vi "Meas Result Get Readings.vi"(5 "table ref":refnum<vi>, 8 "error in (no error)":errorcluster, 9 "ring spot":refnum<vi>, 10 "ring phase":refnum<vi>, 11 "result":T3) -> (0 "error out":errorcluster, 1 "sweep spot index":u16, 2 "phase index":u16, 3 "readings":T1, 4 "quantities":T2)   [LabVIEW 2020]
doc: "Gets readings for selected sweep spot."
uses:
  Meas Results.ctl
  bridge/Bridge Frequency Readings Data.ctl
  drivers/TWM client/Meas Proc QWTB Spectrum Data.ctl
  drivers/TWM client/TWM Phase Info.ctl
  Meas Quantity Names.ctl
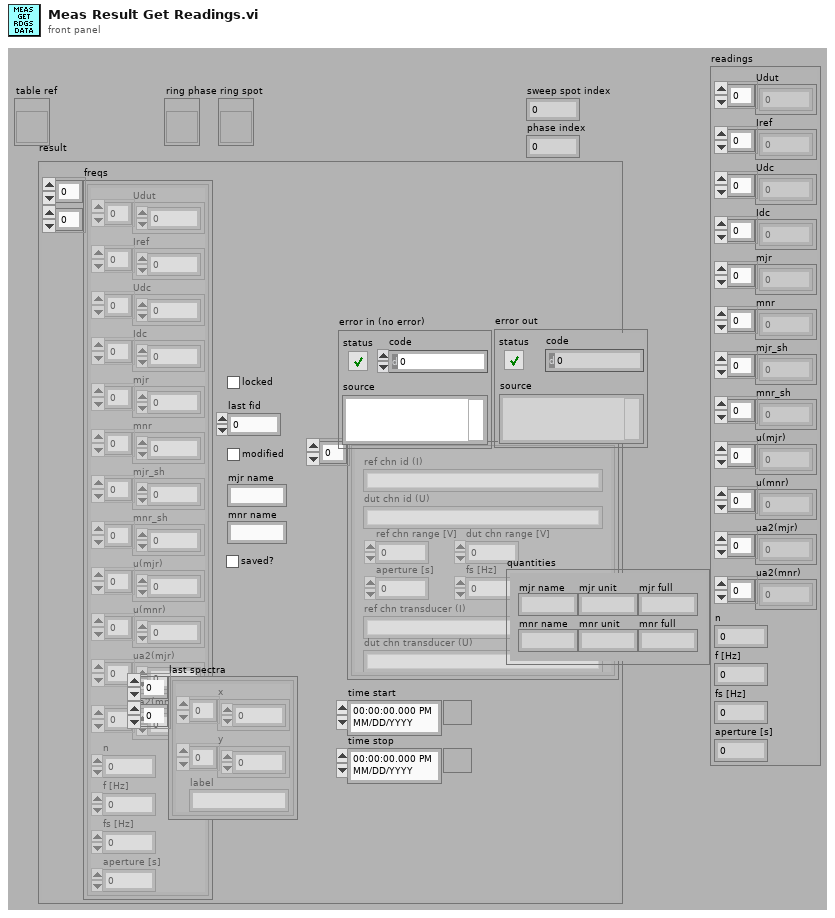
[diagram p1: front panel]
types:
  T1 = typedef "Bridge Frequency Readings Data.ctl" = cluster{"Udut":dbl[], "Iref":dbl[], "Udc":dbl[], "Idc":dbl[], "mjr":dbl[], "mnr":dbl[], "mjr_sh":dbl[], "mnr_sh":dbl[], "u(mjr)":dbl[], "u(mnr)":dbl[], "ua2(mjr)":dbl[], "ua2(mnr)":dbl[], "n":i32, "f [Hz]":dbl, "fs [Hz]":dbl, "aperture [s]":dbl}
  T2 = typedef "Meas Quantity Names.ctl" = cluster{"mjr name":string, "mnr name":string, "mjr unit":string, "mnr unit":string, "mjr full":string, "mnr full":string}
  T3 = typedef "Meas Results.ctl" = cluster{"freqs":T1[][], "locked":bool, "last fid":i32, "modified":bool, "mjr name":string, "mnr name":string, "last spectra":T4[][], "saved?":bool, "TWM phase":T5[], "time start":timestamp, "time stop":timestamp}
  T4 = typedef "Meas Proc QWTB Spectrum Data.ctl" = cluster{"x":sgl[], "y":sgl[], "label":string}
  T5 = typedef "TWM Phase Info.ctl" = cluster{"ref chn id (I)":string, "dut chn id (U)":string, "ref chn range [V]":dbl, "dut chn range [V]":dbl, "aperture [s]":dbl, "fs [Hz]":dbl, "ref chn transducer (I)":string, "dut chn transducer (U)":string}
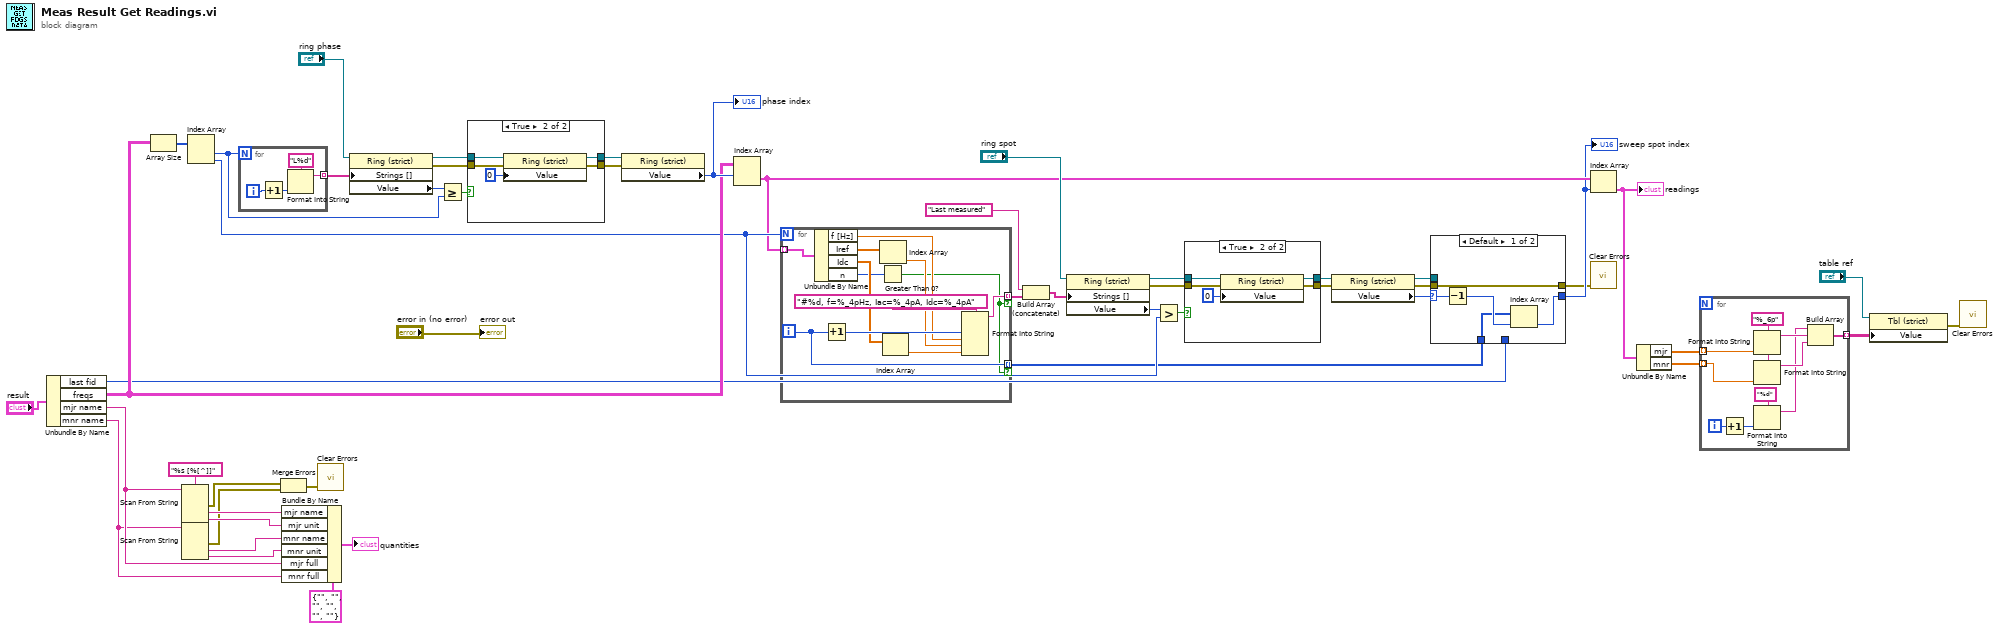
[diagram p0: block diagram]
diagram:
  w47 = "%s [%[^]]" ("format string")
  n1 = Unbundle By Name("result") -> ("last fid"=w3:i32, "freqs"=w27:T1[][], "mjr name"=w44:string, "mnr name"=w43:string)
  n2 = Array Size(array=w27) -> (size(s)=w38:i32[])
  n3 = Scan From String(format string=w47, input string=w44) -> (error out=w40:errorcluster, output 1=w49:string, output 2=w48:string)  [unwired: 4 in, 2 out]
  n4 = Scan From String(format string=w47, input string=w43) -> (error out=w41:errorcluster, output 1=w46:string, output 2=w45:string)  [unwired: 4 in, 2 out]
  n5 = Index Array(array=w38) -> (element #1=w34:i32, element #2=w24:i32)  [unwired: 2 in]
  n6 = for {
    N: w34 -> [_]
    tunnel: [w52] -> w36 mode=indexing
    i -> [w53]
    n7 = Increment(x=w53) -> (x+1=w54:i32)
    n8 = Format Into String(format string="L%d", w54) -> (resulting string=w52:string)  [unwired: 2 in, 1 out]
  }
  n9 = Merge Errors(w40, w41) -> (w39:errorcluster)
  n10 = Bundle By Name(cluster=T2 {"mjr name"="", "mnr name"="", "mjr unit"="", "mnr unit"="", "mjr full"="", "mnr full"=""} ("quantities"), "mjr name"=w49, "mjr unit"=w48, "mnr name"=w46, "mnr unit"=w45, "mjr full"=w44, "mnr full"=w43) -> (→"quantities":T2)
  n11 = call <vilib>:"Clear Errors.vi"("error in (no error)"=w39) -> ()  [unwired: 5 in, 2 out]
  n12 = property class="Ring (strict)"(reference="ring phase", "Strings []"=w36) -> (reference out=w32:refnum<vi>, error out=w30:errorcluster, "Value"=w35:u16)  [unwired: 1 in]
  n13 = Greater Or Equal?(x=w35, y=w34) -> (x >= y?=w33:bool)
  n14 = case shown="True" w33 {
    tunnel: w32 -> [w57 w62]
    tunnel: [w57 w60] -> w31
    tunnel: [w56 w58] -> w29
    tunnel: w30 -> [w56 w59]
    frame False {
    }
    frame True {
      n15 = property class="Ring (strict)"(reference=w62, error in=w59, "Value"=u16 0) -> (reference out=w60:refnum<vi>, error out=w58:errorcluster)
    }
  }
  n16 = property class="Ring (strict)"(reference=w31, error in=w29) -> ("Value"=w28:u16)  [unwired: 2 out]
  "phase index" <- w28
  n17 = Index Array(array=w27, index (row)=w28) -> (element=w16:T1[])  [unwired: 1 in]
  n18 = for {
    N: w24 -> [_]
    tunnel: [w72] -> w8 mode=indexing if=w63
    tunnel: w16 -> [w71] mode=indexing
    tunnel: [w64] -> w1 mode=indexing if=w63
    i -> [w64]
    n19 = Unbundle By Name(w71) -> ("f [Hz]"=w70:dbl, "Iref"=w69:dbl[], "Idc"=w67:dbl[], "n"=w65:i32)
    n20 = Increment(x=w64) -> (x+1=w73:i32)
    n21 = Index Array(array=w69) -> (element=w68:dbl)  [unwired: 1 in]
    n22 = Greater Than 0?(x=w65) -> (x > 0?=w63:bool)
    n23 = Index Array(array=w67) -> (element=w66:dbl)  [unwired: 1 in]
    n24 = Format Into String(format string="#%d, f=%_4pHz, Iac=%_4pA, Idc=%_4pA", w73, w70, w68, w66) -> (resulting string=w72:string)  [unwired: 2 in, 1 out]
  }
  n25 = Build Array (concatenate)("Last measured", w8) -> (w7:string[])
  n26 = property class="Ring (strict)"(reference="ring spot", "Strings []"=w7) -> (reference out=w22:refnum<vi>, error out=w23:errorcluster, "Value"=w25:u16)  [unwired: 1 in]
  n27 = Greater?(x=w25, y=w24) -> (0:w21:bool)
  n28 = case shown="True" w21 {
    tunnel: w22 -> [w76 w81]
    tunnel: [w76 w79] -> w19
    tunnel: [w75 w77] -> w20
    tunnel: w23 -> [w75 w78]
    frame False {
    }
    frame True {
      n29 = property class="Ring (strict)"(reference=w81, error in=w78, "Value"=u16 0) -> (reference out=w79:refnum<vi>, error out=w77:errorcluster)
    }
  }
  n30 = property class="Ring (strict)"(reference=w19, error in=w20) -> (reference out=w17:refnum<vi>, error out=w18:errorcluster, "Value"=w4:u16)
  n31 = case shown="Default" w4 {
    selector: w4 -> [w86 _]
    tunnel: w18 -> [w85 w87]
    tunnel: w17 -> [_ _]
    tunnel: [w83 w88] -> w15
    tunnel: w3 -> [_ w88]
    tunnel: [w85 w87] -> w2
    tunnel: w1 -> [w82 _]
    frame Default {
      n32 = Decrement(x=w86) -> (x-1=w84:u16)
      n33 = Index Array(array=w82, index=w84) -> (element=w83:i32)
    }
    frame 0 {
    }
  }
  "sweep spot index" <- w15
  n34 = Index Array(array=w16, index=w15) -> (element=w14:T1)
  "readings" <- w14
  n35 = call <vilib>:"Clear Errors.vi"("error in (no error)"=w2) -> ()  [unwired: 5 in, 2 out]
  n36 = Unbundle By Name(w14) -> ("mjr"=w13:dbl[], "mnr"=w12:dbl[])
  n37 = for {
    tunnel: w13 -> [w94] mode=indexing
    tunnel: w12 -> [w93] mode=indexing
    tunnel: [w89] -> w10 mode=indexing
    i -> [w98]
    w95 = "%_6p" ("format string")
    n38 = Increment(x=w98) -> (x+1=w96:i32)
    n39 = Format Into String(format string=w95, w94) -> (resulting string=w92:string)  [unwired: 2 in, 1 out]
    n40 = Format Into String(format string=w95, w93) -> (resulting string=w91:string)  [unwired: 2 in, 1 out]
    n41 = Format Into String(format string="%d", w96) -> (resulting string=w90:string)  [unwired: 2 in, 1 out]
    n42 = Build Array(w90, w92, w91) -> (w89:string[])
  }
  n43 = property class="Tbl (strict)"(reference="table ref", "Value"=w10) -> (error out=w9:errorcluster)  [unwired: 1 in, 1 out]
  n44 = call <vilib>:"Clear Errors.vi"("error in (no error)"=w9) -> ()  [unwired: 5 in, 2 out]
  "error out" <- "error in (no error)"
